vi "Run.vi"(8 "error in (no error)":errorcluster caption="entrée d'erreur (pas d'erreur)", 11 "Multilabel_Classification.lvclass":refnum<class "Multilabel_Classification.lvclass">) -> (0 "error out":errorcluster caption="sortie d'erreur", 2 "Data":T1, 3 "Multilabel_Classification.lvclass":refnum<class "Multilabel_Classification.lvclass">)   [LabVIEW 2020, in "Multilabel_Classification.lvclass"]
doc: "Returns : \n\nX : array of shape [n_samples, n_features]\nThe generated samples.\n\nY : array or sparse CSR matrix of shape [n_samples, n_classes]\nThe label sets.\n\np_c : array, shape [n_classes]\nThe probability of each class being drawn. Only returned if return_distributions=True.\n\np_w_c : array, shape [n_features, n_classes]\nThe probability of each feature being drawn given each class. Only returned if return_distributions=True."
uses:
  Multilabel_Classification.lvclass
  Multilabel_Classification.lvclass/Multilabel_Classification.ctl
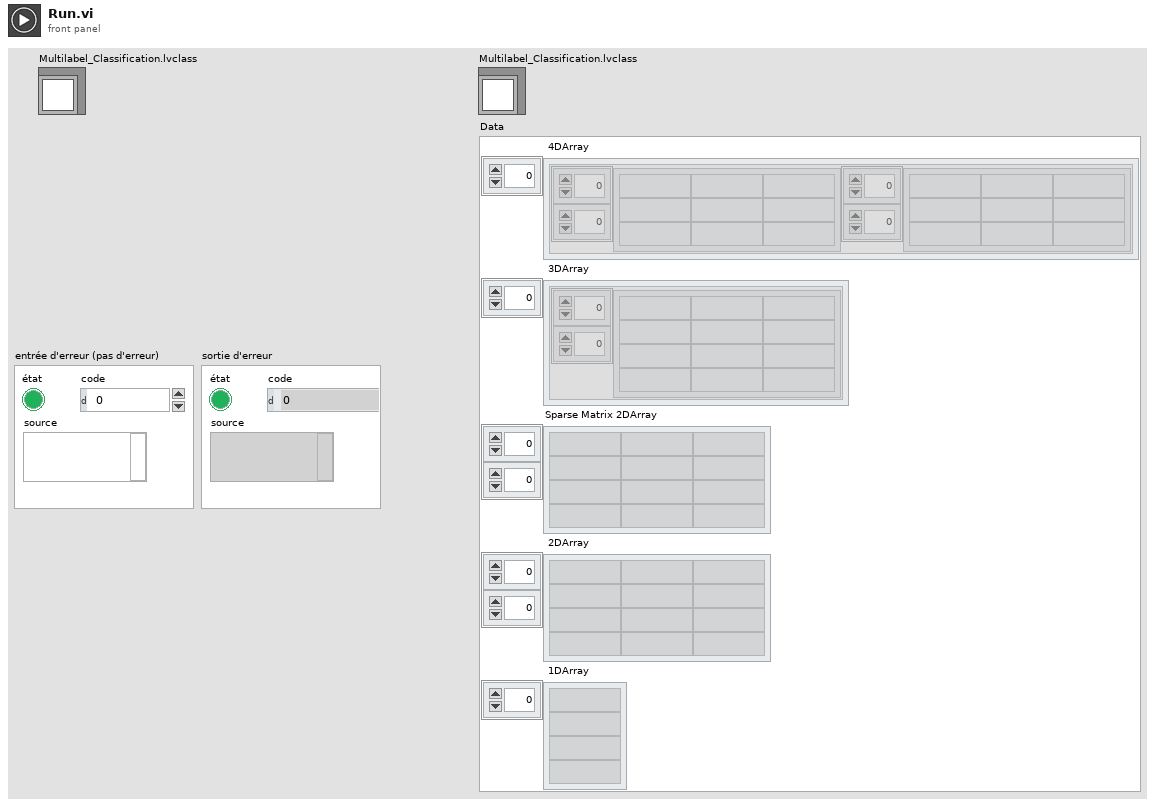
[diagram p1: front panel]
types:
  T1 = cluster{" 4DArray":cluster{"1":string[][], "2":string[][]}[], " 3DArray":cluster{"Tableau":string[][]}[], "Sparse Matrix 2DArray":string[][], " 2DArray":string[][], " 1DArray":string[]}
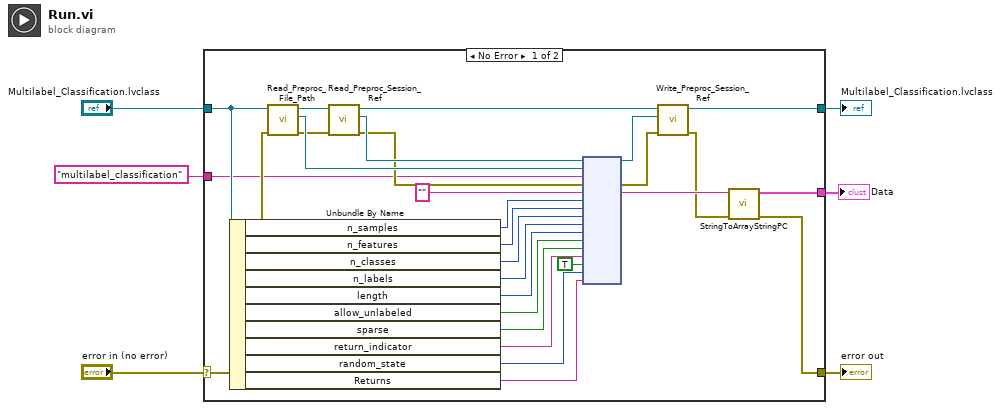
[diagram p0: block diagram]
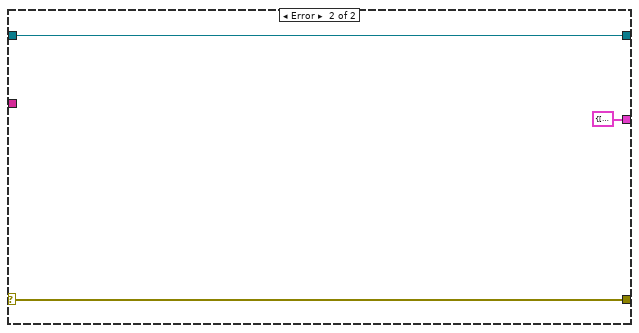
[diagram p2: hidden frame]
diagram:
  n1 = case shown="No Error" "error in (no error)" {
    selector: "error in (no error)" -> [w23 w37]
    tunnel: [w8 w37] -> w5
    tunnel: [w11 w36] -> w3
    tunnel: "Multilabel_Classification.lvclass" -> [w22 w36]
    tunnel: "multilabel_classification" -> [w21 _]
    tunnel: [w7 T1 {" 4DArray"=[], " 3DArray"=[], "Sparse Matrix 2DArray"=[], " 2DArray"=[], " 1DArray"=[]} ("Data")] -> w1
    frame No Error {
      n2 = Unbundle By Name(w22) -> ("n_samples"=w25:u32, "n_features"=w24:u32, "n_classes"=w20:u32, "n_labels"=w19:u32, "length"=w18:u32, "allow_unlabeled"=w17:bool, "sparse"=w16:bool, "return_indicator"=w15:string, "random_state"=w13:i32, "Returns"=w12:string)
      n3 = call-dynamic "Read_Preproc_File_Path.vi"("error in (no error)"=w23, "Python in"=w22) -> ("error out"=w29:errorcluster, "File_Path"=w32:path, "Python out"=w34:refnum<class "Multilabel_Classification.lvclass">)  [unwired: 7 in]
      n4 = call-dynamic "Read_Preproc_Session_Ref.vi"("error in (no error)"=w29, "Python in"=w34) -> ("error out"=w30:errorcluster, "Session_ref"=w31:refnum<k35>, "Python out"=w33:refnum<class "Multilabel_Classification.lvclass">)  [unwired: 7 in]
      n5 = node(w31, w32, w21, w30, "", w25, w24, w20, w19, w18, w17, w16, w15, TRUE, w13, w12) -> (w26:refnum<k35>, w28:errorcluster, w10:string)  [unwired: 11 in, 2 out]
      n6 = call-dynamic "Write_Preproc_Session_Ref.vi"("error in (no error)"=w28, "Session_ref"=w26, "Python in"=w33) -> ("error out"=w9:errorcluster, "Python out"=w11:refnum<class "Multilabel_Classification.lvclass">)  [unwired: 7 in]
      n7 = call "StringToArrayStringPC.vi"("sortie d'erreur"=w9, "Return value"=w10) -> ("sortie d'erreur"=w8:errorcluster, "Data"=w7:T1)  [unwired: 8 in]
    }
    frame Error {
    }
  }
  "error out" <- w5
  "Multilabel_Classification.lvclass" <- w3
  "Data" <- w1
